vi "play ground.vi"() -> ()   [LabVIEW 2013]
panel:
  out "最小值":dbl
  out "最大值":dbl
  out "大小":i32
  out "波形图":dbl[](graph)
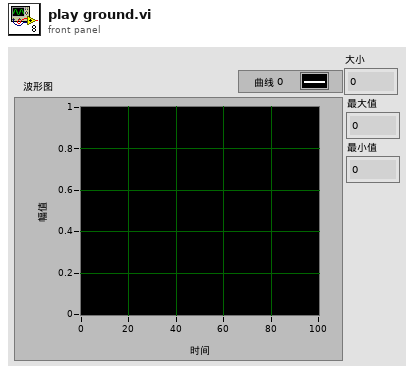
[diagram p1: front panel]
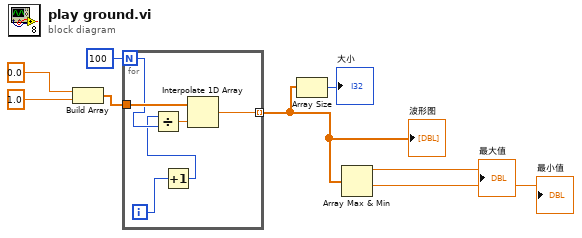
[diagram p0: block diagram]
diagram:
  n1 = Build Array(0.0 ("元素"), 1.0 ("元素")) -> (w6:dbl[])
  n2 = for {
    N: 100 -> [w12]
    tunnel: w6 -> [w14]
    tunnel: [w11] -> w3 mode=indexing
    i -> [w10]
    n3 = Increment(x=w10) -> (x+1=w9:i32)
    n4 = Divide(x=w9, y=w12) -> (x/y=w13:dbl)
    n5 = Interpolate 1D Array(1:w13, 2:w14) -> (0:w11:dbl)
  }
  "波形图" <- w3
  n6 = Array Size(array=w3) -> (size(s)=→"大小":i32)
  n7 = Array Max & Min(array=w3) -> (max value=→"最大值":dbl, min value=→"最小值":dbl)  [unwired: 2 out]
